vi "START.vi"() -> (0 "number":u32)   [LabVIEW 2014]
panel:
  in  "?":cluster{"OK Button":bool, "OK Button 2":bool}
  # "MODE :"
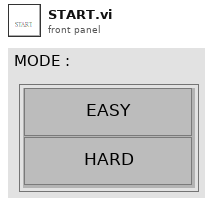
[diagram p1: front panel]
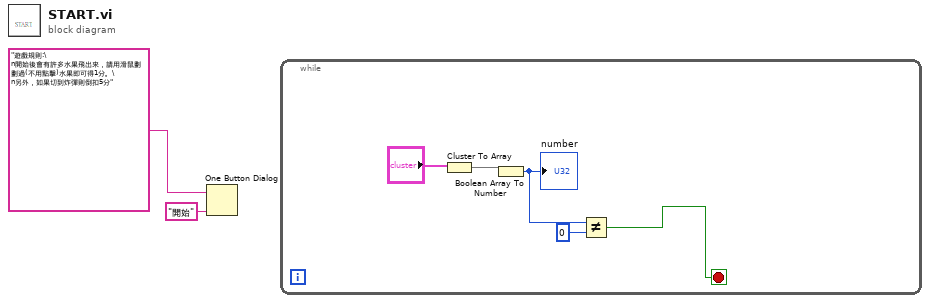
[diagram p0: block diagram]
diagram:
  n1 = One Button Dialog(message="遊戲規則:\n開始後會有許多水果飛出來，請用滑鼠劃劃過(不用點擊)水果即可得1分。\n另外，如果切到炸彈則倒扣5分", button name ("OK")="開始") -> ()  [unwired: 1 out]
  n2 = while {
    stop <- w3 stop-if-true
    n3 = Cluster To Array(cluster="?") -> (array=w6:bool[])
    n4 = Boolean Array To Number(Boolean array=w6) -> (number=w5:u32)
    "number" <- w5
    n5 = Not Equal?(x=w5, y=u32 0) -> (x != y?=w3:bool)
  }
